vi "OEE Calculator.vi"(8 "Total T":u32, 9 "Shift  wise DT":u32, 10 "Pass":dbl, 11 "Total":dbl) -> (0 "Performance":dbl, 1 "Avilability":dbl, 2 "Qulity":dbl format="%#_3g", 3 "OEE":dbl format="%#.3g")   [LabVIEW 2017]
panel:
  out "Run Time":u32
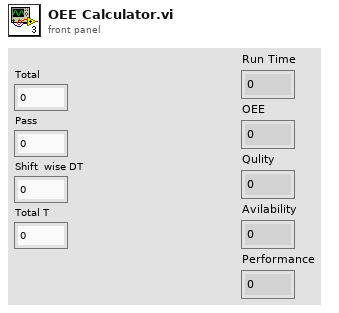
[diagram p1: front panel]
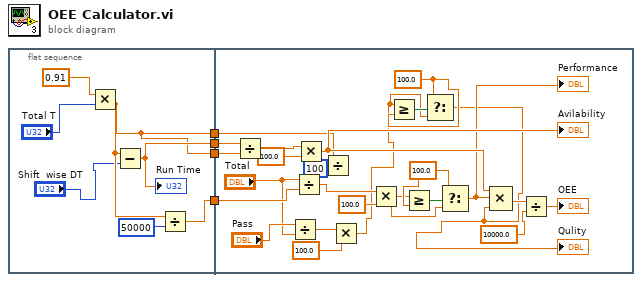
[diagram p0: block diagram]
diagram:
  n1 = flat-sequence {
    tunnel: [w11] -> w4
    tunnel: [w8] -> w3
    tunnel: [w8] -> w2
    tunnel: [w9] -> w1
    tunnel: w4 -> [w26]
    tunnel: w3 -> [w36]
    tunnel: w2 -> [w24]
    tunnel: w1 -> [w22]
    frame #0 {
      n2 = Multiply(x=0.91 ("y"), y="Total T") -> (x*y=w8:dbl)
      n3 = Subtract(x=w8, y="Shift  wise DT") -> (x-y=w11:dbl)
      "Run Time" <- w11
      n4 = Divide(x=w8, y=u32 50000) -> (x/y=w9:dbl)
    }
    frame #1 {
      w16 = 100.0 ("t")
      w20 = 100.0 ("t")
      n5 = Divide(x=w26, y=w36) -> (x/y=w35:dbl)
      n6 = Divide(x="Pass", y="Total") -> (x/y=w33:dbl)
      n7 = Divide(x="Total", y=w22) -> (x/y=w25:dbl)
      n8 = Multiply(x=w35, y=100.0) -> (x*y=w27:dbl)
      "Avilability" <- w27
      n9 = Divide(x=w24, y=u32 100) -> ()  [unwired: 1 out]
      n10 = Multiply(x=w33, y=100.0) -> (x*y=w15:dbl)
      n11 = Multiply(x=w25, y=100.0) -> (x*y=w19:dbl)
      n12 = Greater Or Equal?(x=w15, y=w16) -> (x >= y?=w17:bool)
      n13 = Greater Or Equal?(x=w19, y=w20) -> (x >= y?=w21:bool)
      n14 = Select(t=w16, s=w17, f=w15) -> (s? t:f=w14:dbl)
      "Qulity" <- w14
      n15 = Select(t=w20, s=w21, f=w19) -> (s? t:f=w18:dbl)
      "Performance" <- w18
      n16 = Compound Arithmetic op=MULTIPLY(w27, w18, w14) -> (w30:dbl)
      n17 = Divide(x=w30, y=10000.0) -> (x/y=→"OEE":dbl)
    }
  }
